vi "reset_run_button.vi"(6 "error in":errorcluster, 9 "Front panel references":T1) -> (0 "error out":errorcluster)   [LabVIEW 2010]
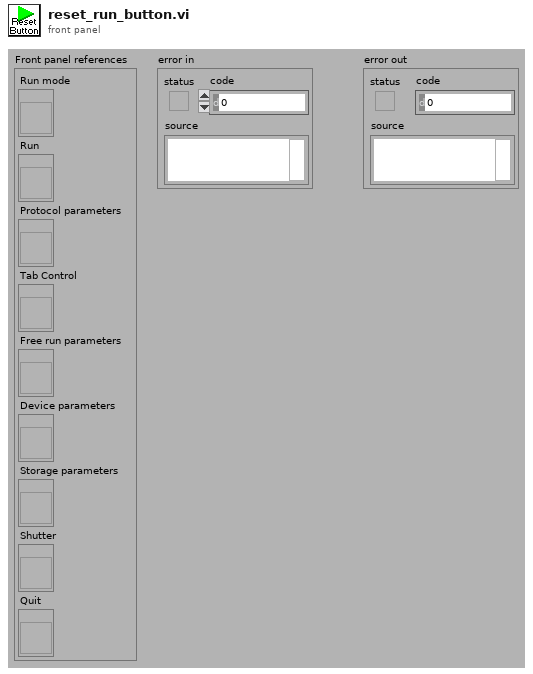
[diagram p1: front panel]
types:
  T1 = cluster{"Run mode":refnum<vi>, "Run":refnum<vi>, "Protocol parameters":refnum<vi>, "Tab Control":refnum<vi>, "Free run parameters":refnum<vi>, "Device parameters":refnum<vi>, "Storage parameters":refnum<vi>, "Shutter":refnum<vi>, "Quit":refnum<vi>}
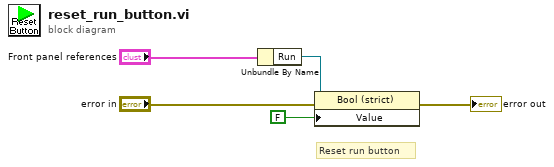
[diagram p0: block diagram]
diagram:
  # "Reset run button"
  n1 = Unbundle By Name("Front panel references") -> ("Run"=w2:refnum<vi>)
  n2 = property class="Bool (strict)"(reference=w2, error in="error in", "Value"=FALSE ("Run")) -> (error out=→"error out":errorcluster)  [unwired: 1 out]
